vi "ASYNC_Adam_client.vi"(2 "Values":dbl[](array[numeric]) format="%.2f", 3 "Check Value is in the scan table?":bool, 4 "Channel Names":string[](array[string])) -> (0 "Scan Comments":string[](array[string]), 1 "Calibrated Units":dbl[](array[numeric]) format="%.4f")   [LabVIEW 2014]
uses:
  Anemometry/Anemometry Sub Vis/Controls/Global_mode.ctl
  Sub VIs/ADAM Controls/Update_scan_value.ctl
  Anemometry/Anemometry Sub Vis/Globals/Preference_global.vi
panel:
  out "Iterations":i32
  in  "ASYNC Adam server":refnum<vi>
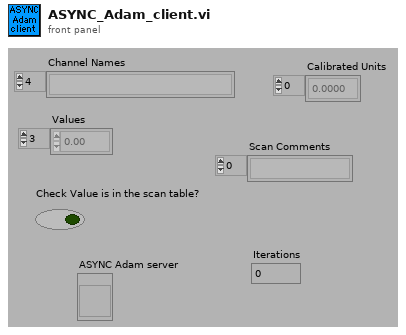
[diagram p1: front panel]
types:
  T1 = typedef "Server_Comms.ctl" = enum16{"Server Link Healthy", "Do Not Link To Server"}
  T2 = typedef "Update_scan_value.ctl" = cluster{"Channel Name":string, "New Value":dbl}
  T3 = typedef "Global_mode.ctl" = enum16{"Read Global", "Load Global From File", "Write Global to File"}
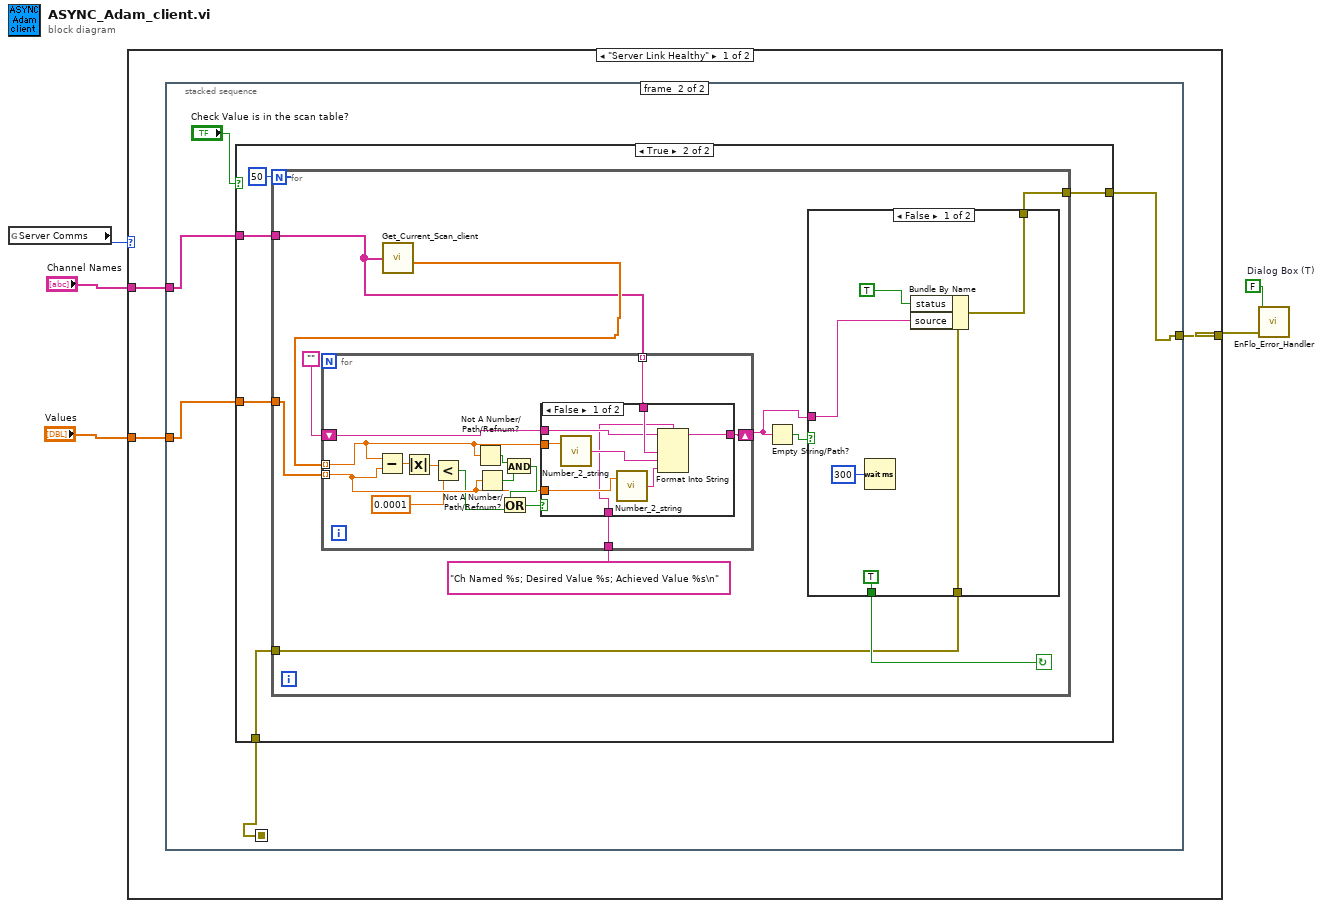
[diagram p0: block diagram]
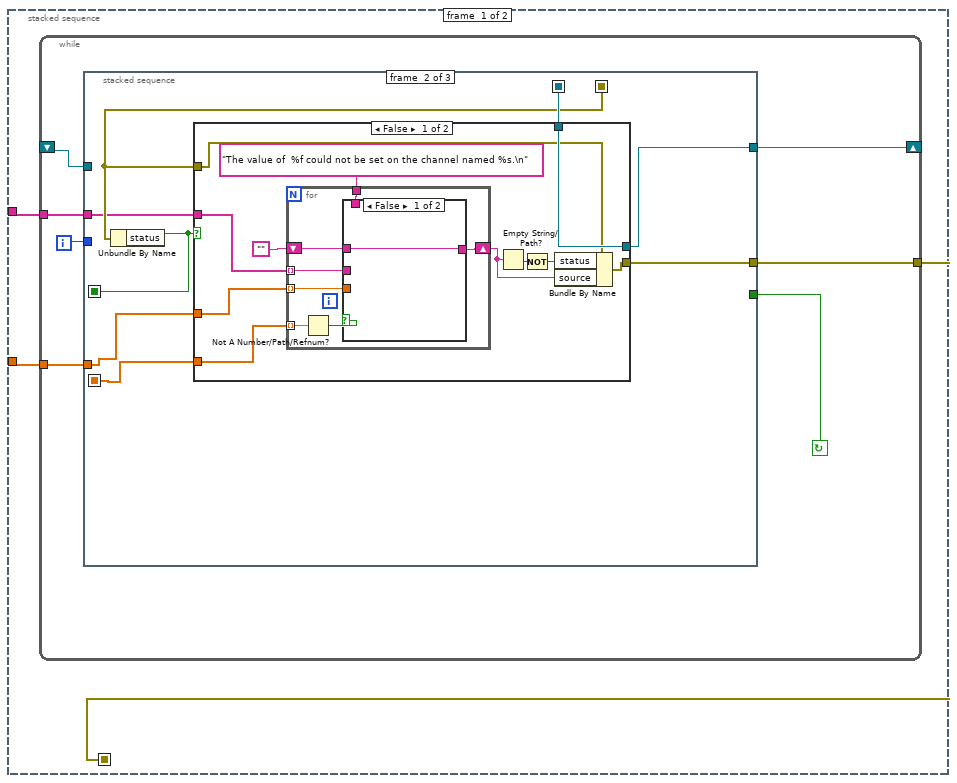
[diagram p2: hidden frame]
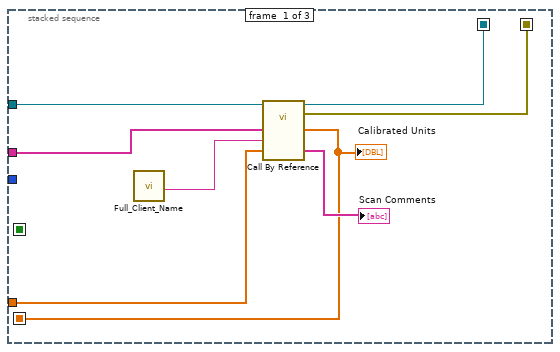
[diagram p3: hidden frame]
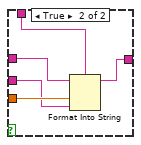
[diagram p4: hidden frame]
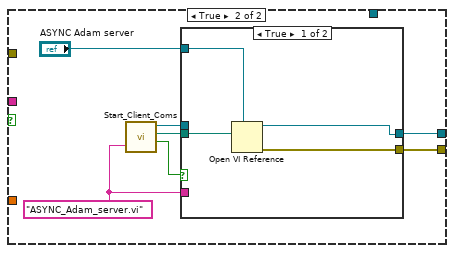
[diagram p5: hidden frame]
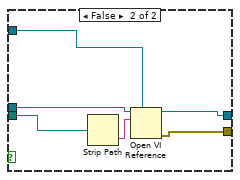
[diagram p6: hidden frame]
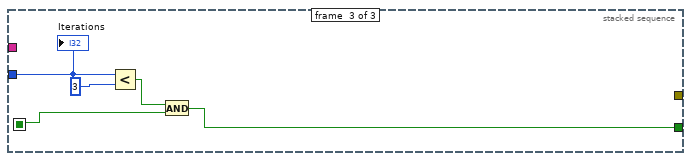
[diagram p7: hidden frame]
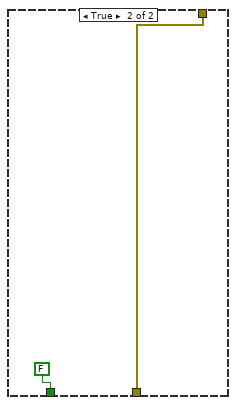
[diagram p10: hidden frame]
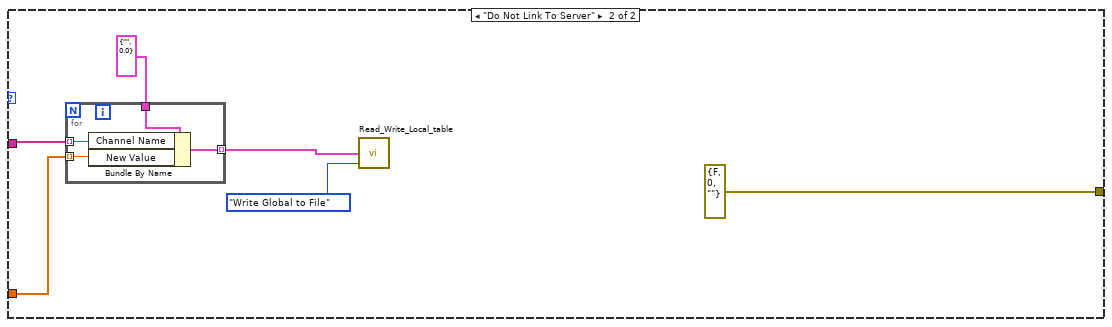
[diagram p11: hidden frame]
diagram:
  w1 = FALSE  # Dialog Box (T)
  n1 = global read "Preference_global.vi" "Server Comms"() -> (w4:T1)
  n2 = case shown="\"Server Link Healthy\"" w4 {
    tunnel: [w8 errorcluster {"status"=FALSE, "code"=0, "source"=""}] -> w5
    tunnel: "Channel Names" -> [w7 w135]
    tunnel: "Values" -> [w6 w134]
    frame "Server Link Healthy" {
      n3 = stacked-sequence {
        seq-local: [w9 _] -> [_ w82]
        tunnel: [_ w81] -> w8
        tunnel: w7 -> [w11 w84]
        tunnel: w6 -> [w10 w83]
        frame #0 {
          n4 = while {
            tunnel: w10 -> [w12]
            tunnel: w11 -> [w13]
            tunnel: [w14] -> w9
            shift-left: _ -> [w18]
            shift-right: [w17] -> _
            i -> [w16]
            stop <- w15 continue-if-true
            n5 = stacked-sequence {
              seq-local: [w24 _ _] -> [_ w34 _]
              seq-local: [w26 _ _] -> [_ w32 _]
              seq-local: [_ w33 _] -> [_ _ w77]
              seq-local: [w19 _ _] -> [_ w30 _]
              tunnel: w18 -> [w25 _ _]
              tunnel: [_ w31 _] -> w17
              tunnel: w16 -> [_ _ w78]
              tunnel: [_ _ w76] -> w15
              tunnel: [_ w27 _] -> w14
              tunnel: w13 -> [w22 w28 _]
              tunnel: w12 -> [w21 w29 _]
              frame #0 {
                n6 = call "Full_Client_Name.vi"() -> ("Client Name"=w20:string)
                n7 = call-by-ref "?"(reference=w25, "Values"=w21, "Client HD name"=w20, "Channel Names"=w22) -> (reference out=w24:refnum<vi>, error out=w26:errorcluster, "Scan Comments"=→"Scan Comments":string[], "Calibrated Units"=w19:dbl[])  [unwired: 2 in]
                "Calibrated Units" <- w19
              }
              frame #1 {
                n8 = Unbundle By Name(w32) -> ("status"=w33:bool)
                n9 = case shown="False" w33 {
                  tunnel: w34 -> [w45 _]
                  tunnel: [w38 w62] -> w27
                  tunnel: w32 -> [w39 _]
                  tunnel: [w45 w61] -> w31
                  tunnel: w30 -> [w44 _]
                  tunnel: w29 -> [w43 _]
                  tunnel: w28 -> [w42 _]
                  frame False {
                    n10 = for {
                      shift-right: [w47] -> w35
                      shift-left: "" -> [w48]
                      tunnel: w44 -> [w52] mode=indexing
                      tunnel: w43 -> [w50] mode=indexing
                      tunnel: w42 -> [w49] mode=indexing
                      tunnel: "The value of  %f could not be set on the channel named %s.\n" ("format string") -> [w46]
                      n11 = Not A Number/Path/Refnum?(number/path/refnum=w52) -> (NaN/Path/Refnum?=w51:bool)
                      n12 = case shown="False" w51 {
                        tunnel: w50 -> [_ w58]
                        tunnel: w49 -> [_ w57]
                        tunnel: w48 -> [w53 w56]
                        tunnel: [w53 w55] -> w47
                        tunnel: w46 -> [_ w54]
                        frame False {
                        }
                        frame True {
                          n13 = Format Into String(format string=w54, initial string=w56, w58, w57) -> (resulting string=w55:string)  [unwired: 1 in, 1 out]
                        }
                      }
                    }
                    n14 = Empty String/Path?(string/path=w35) -> (empty?=w37:bool)
                    n15 = Not(x=w37) -> (.not. x?=w36:bool)
                    n16 = Bundle By Name(cluster=w39, "status"=w36, "source"=w35) -> (w38:errorcluster)
                  }
                  frame True {
                    w60 = "ASYNC_Adam_server.vi"
                    n17 = call "Start_Client_Coms.vi"("VI name to run on server"=w60) -> ("LabVIEW application reference"=w65:refnum<vi>, "Checked VI name"=w63:path, "Local Call"=w64:bool)  [unwired: 1 in, 1 out]
                    n18 = case shown="True" w64 {
                      tunnel: w63 -> [w69 w72]
                      tunnel: w65 -> [_ w70]
                      tunnel: [w68 w73] -> w62
                      tunnel: [w67 w74] -> w61
                      tunnel: w60 -> [_ _]
                      tunnel: "ASYNC Adam server" -> [w66 w71]
                      frame True {
                        n19 = Open VI Reference(type specifier VI Refnum (for type only)=w66, vi path=w69) -> (vi reference=w67:refnum<vi>, error out=w68:errorcluster)  [unwired: 1 in, 3 out]
                      }
                      frame False {
                        n20 = Strip Path(path=w72) -> (name=w75:string)  [unwired: 1 out]
                        n21 = Open VI Reference(type specifier VI Refnum (for type only)=w71, application reference (local)=w70, vi path=w75) -> (vi reference=w74:refnum<vi>, error out=w73:errorcluster)  [unwired: 1 in, 2 out]
                      }
                    }
                  }
                }
              }
              frame #2 {
                n22 = Less?(x=w78, y=3) -> (x < y?=w80:bool)
                n23 = And(x=w80, y=w77) -> (x .and. y?=w76:bool)
                "Iterations" <- w78
              }
            }
          }
        }
        frame #1 {
          n24 = case shown="True" "Check Value is in the scan table?" {
            tunnel: w84 -> [_ w90]
            tunnel: w83 -> [_ w89]
            tunnel: w82 -> [w86 w88]
            tunnel: [w86 w87] -> w81
            frame False {
            }
            frame True {
              n25 = for {
                N: 50 -> [_]
                tunnel: w90 -> [w97]
                tunnel: w89 -> [w98]
                tunnel: [w93] -> w87
                tunnel: w88 -> [w92]
                stop <- w94 continue-if-true
                n26 = call "Get_Current_Scan_client.vi"("ADAM Ch Names"=w97) -> ("Numerical Values"=w99:dbl[])  [unwired: 3 out]
                n27 = for {
                  shift-right: [w114] -> w95
                  shift-left: "" -> [w113]
                  tunnel: w98 -> [w106] mode=indexing
                  tunnel: w99 -> [w107] mode=indexing
                  tunnel: "Ch Named %s; Desired Value %s; Achieved Value %s\n" ("format string") -> [w115]
                  tunnel: w97 -> [w108] mode=indexing
                  n28 = Subtract(x=w107, y=w106) -> (x-y=w105:dbl)
                  n29 = Absolute Value(x=w105) -> (abs(x)=w104:dbl)
                  n30 = Less?(x=w104, y=0.0001) -> (x < y?=w102:bool)
                  n31 = Not A Number/Path/Refnum?(number/path/refnum=w107) -> (NaN/Path/Refnum?=w110:bool)
                  n32 = Not A Number/Path/Refnum?(number/path/refnum=w106) -> (NaN/Path/Refnum?=w111:bool)
                  n33 = And(x=w110, y=w111) -> (x .and. y?=w109:bool)
                  n34 = Or(x=w109, y=w102) -> (x .or. y?=w112:bool)
                  n35 = case shown="False" w112 {
                    tunnel: w108 -> [w123 _]
                    tunnel: w107 -> [w117 _]
                    tunnel: w106 -> [w118 _]
                    tunnel: w115 -> [w116 _]
                    tunnel: [w122 w124] -> w114
                    tunnel: w113 -> [w121 w124]
                    frame False {
                      n36 = call "Number_2_string.vi"("number"=w117) -> ("String"=w119:string)  [unwired: 1 in]
                      n37 = call "Number_2_string.vi"("number"=w118) -> ("String"=w120:string)  [unwired: 1 in]
                      n38 = Format Into String(format string=w116, initial string=w121, w123, w119, w120) -> (resulting string=w122:string)  [unwired: 1 in, 1 out]
                    }
                    frame True {
                    }
                  }
                }
                n39 = Empty String/Path?(string/path=w95) -> (empty?=w96:bool)
                n40 = case shown="False" w96 {
                  tunnel: [TRUE FALSE] -> w94
                  tunnel: w95 -> [w130 _]
                  tunnel: [w129 w131] -> w93
                  tunnel: w92 -> [w128 w131]
                  frame False {
                    n41 = Wait (ms)(milliseconds to wait=u32 300) -> ()  [unwired: 1 out]
                    n42 = Bundle By Name(cluster=w128, "status"=TRUE, "source"=w130) -> (w129:errorcluster)
                  }
                  frame True {
                  }
                }
              }
            }
          }
        }
      }
    }
    frame "Do Not Link To Server" {
      n43 = for {
        tunnel: T2 {"Channel Name"="", "New Value"=0.0} ("Update Scan Value Cluster") -> [w142]
        tunnel: w135 -> [w141] mode=indexing
        tunnel: w134 -> [w140] mode=indexing
        tunnel: [w139] -> w133 mode=indexing
        n44 = Bundle By Name(cluster=w142, "Channel Name"=w141, "New Value"=w140) -> (w139:T2)
      }
      n45 = call "Read_Write_Local_table.vi"("Mode"=Global_mode."Write Global to File", "Ch Values in"=w133) -> ()  [unwired: 1 in, 3 out]
    }
  }
  n46 = call "EnFlo_Error_Handler.vi"("error in (no error)"=w5, "Dialog Box (T)"=w1) -> ()  [unwired: 1 in, 3 out]
